vi "VI Icon Browser.vi"() -> ()   [LabVIEW 2011]
panel:
  out "2D VI Icon":picture[][](array[picture])=[[bytes[1002], bytes[798], bytes[222], bytes[318], bytes[558]], [bytes[1512], bytes[537], bytes[1170], bytes[651], bytes[1170]], [bytes[798], bytes[948], bytes[273], bytes[1101], bytes[420]], [bytes[1065], bytes[462], bytes[705], bytes[1380], bytes[798]], [bytes[756], bytes[534], bytes[2118], bytes[714], bytes[798]], [bytes[810], bytes[1230], bytes[798], bytes[1230], bytes[1218]], [bytes[2118], bytes[525], bytes[3102], bytes[1458], bytes[516]], [bytes[1512], bytes[1161], bytes[300], bytes[537], bytes[1662]], [bytes[654], bytes[2298], bytes[798], bytes[798], bytes[1626]], [bytes[732], bytes[1110], bytes[393], bytes[2130], bytes[798]], [bytes[537], bytes[744], bytes[1353], bytes[1488], bytes[345]], [bytes[798], bytes[2379], bytes[222], bytes[273], bytes[798]], [bytes[798], bytes[705], bytes[2382], bytes[525], bytes[1590]], [bytes[390], bytes[0], bytes[0], bytes[0], bytes[0]]]
  out "1D VI Icon":picture[](array[picture])=[bytes[1002], bytes[798], bytes[222], bytes[318], bytes[558], bytes[1512], bytes[537], bytes[1170], bytes[651], bytes[1170], bytes[798], bytes[948], bytes[273], bytes[1101], bytes[420], bytes[1065], bytes[462], bytes[705], bytes[1380], bytes[798], bytes[756], bytes[534], bytes[2118], bytes[714], bytes[798], bytes[810], bytes[1230], bytes[798], bytes[1230], bytes[1218], bytes[2118], bytes[525], bytes[3102], bytes[1458], bytes[516], bytes[1512], bytes[1161], bytes[300], bytes[537], bytes[1662], bytes[654], bytes[2298], bytes[798], bytes[798], bytes[1626], bytes[732], bytes[1110], bytes[393], bytes[2130], bytes[798], bytes[537], bytes[744], bytes[1353], bytes[1488], bytes[345], bytes[798], bytes[2379], bytes[222], bytes[273], bytes[798], bytes[798], bytes[705], bytes[2382], bytes[525], bytes[1590], bytes[390]]
  in  "停止按钮":bool
  in  "VI Icon":string(combo)="操作"
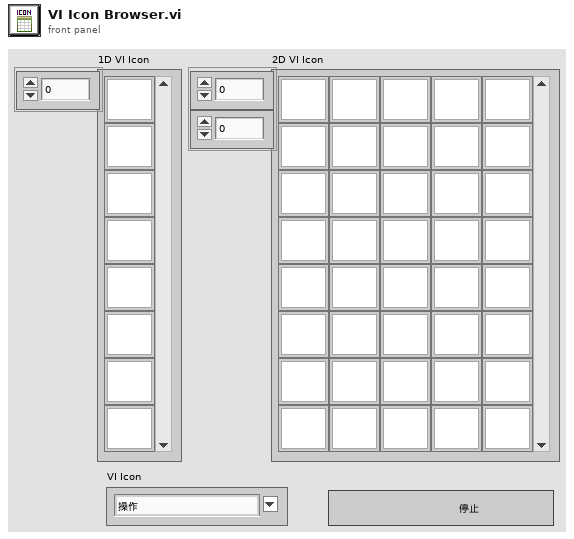
[diagram p1: front panel]
types:
  T1 = typedef "LVBoundsTypeDef.ctl" = cluster{"Width":u32, "Height":u32}
  T2 = typedef "imagedata.ctl" = cluster{"image type":i32, "image depth":i32, "image":u8[], "mask":u8[], "colors":u32[], "Rectangle":cluster{"left":i16, "top":i16, "right":i16, "bottom":i16}}
  T3 = cluster{"left":i16, "top":i16, "right":i16, "bottom":i16}
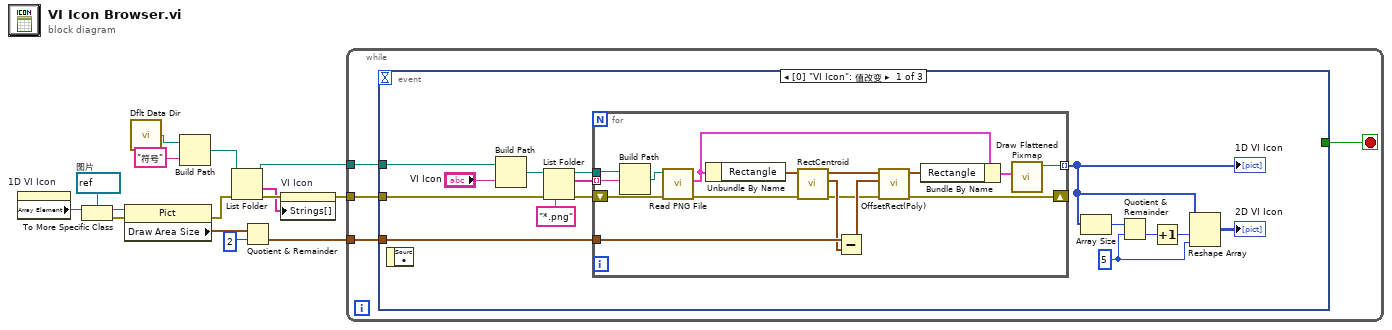
[diagram p0: block diagram]
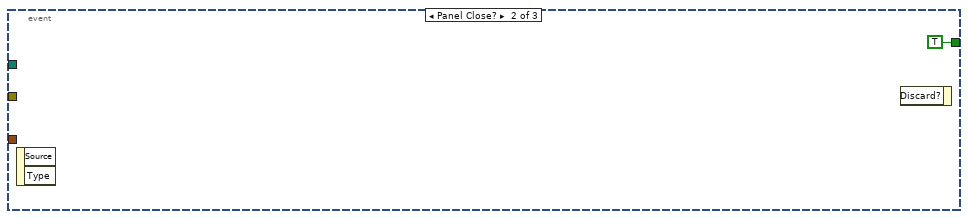
[diagram p2: hidden frame]
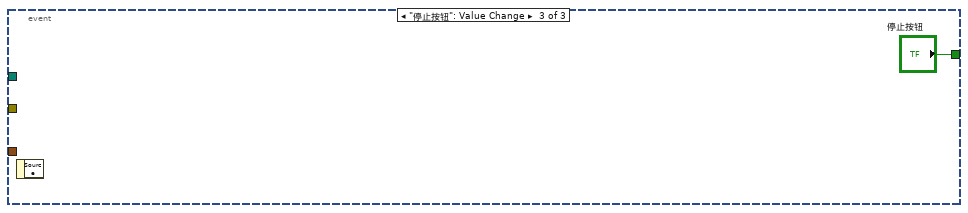
[diagram p3: hidden frame]
diagram:
  w5 = refnum<vi> refnum  # 图片
  n1 = property on="1D VI Icon" class="Arr (严格)"() -> ("Array Element"=w4:refnum<vi>)  [unwired: 2 in, 2 out]
  n2 = To More Specific Class(target class=w5, reference=w4) -> (specific class reference=w6:refnum<vi>, error out=w7:errorcluster)  [unwired: 1 in]
  n3 = property class="Pict"(reference=w6, error in=w7) -> (error out=w1:errorcluster, "Draw Area Size"=w8:T1)  [unwired: 1 out]
  n4 = call <vilib>:"Dflt Data Dir.vi"() -> ("App:Default Data Directory"=w14:path)
  n5 = Build Path(base path=w14, name or relative path="符号" ("名称或相对路径")) -> (appended path=w10:path)
  n6 = List Folder(path=w10, error in=w1) -> (path out=w2:path, folder names=w12:string[], error out=w13:errorcluster)  [unwired: 2 in, 1 out]
  n7 = Quotient & Remainder(x=w8, y=2) -> (floor(x/y)=w3:T1)  [unwired: 1 out]
  n8 = property on="VI Icon" class="CmbBox"(error in=w13, "Strings[]"=w12) -> (error out=w11:errorcluster)  [unwired: 1 in, 1 out]
  n9 = while {
    tunnel: w11 -> [w16]
    tunnel: w2 -> [w18]
    tunnel: w3 -> [w17]
    stop <- w19 stop-if-true
    n10 = event shown="[0] \"VI Icon\": 值改变" {
      selector: _ -> [_ _ _]
      dyn-events: _ -> [_ _ _]
      timeout: _ -> [_ _ _]
      tunnel: [_ TRUE ("停止按钮") "停止按钮"] -> w19
      tunnel: w18 -> [w33 _ _]
      tunnel: w17 -> [w28 _ _]
      tunnel: w16 -> [w21 _ _]
      event "VI Icon": Value Change {
        w22 = 5 ("y")
        n11 = event-data() -> ()  [unwired: 1 in, 1 out]
        n12 = Build Path(base path=w33, name or relative path="VI Icon") -> (appended path=w31:path)
        n13 = List Folder(path=w31, pattern="*.png" ("模式"), error in=w21) -> (path out=w29:path, filenames=w30:string[], error out=w20:errorcluster)  [unwired: 1 in, 1 out]
        n14 = for {
          tunnel: w29 -> [w50]
          tunnel: w30 -> [w49] mode=indexing
          tunnel: [w47] -> w26 mode=indexing
          tunnel: w28 -> [w46]
          shift-right: [w36] -> _
          shift-left: w20 -> [w39]
          n15 = Build Path(base path=w50, name or relative path=w49) -> (appended path=w48:path)
          n16 = call <vilib>:"Read PNG File.vi"("error in (no error)"=w39, "path to PNG file"=w48) -> ("error out"=w38:errorcluster, "image data"=w42:T2)  [unwired: 7 in, 1 out]
          n17 = Unbundle By Name(w42) -> ("Rectangle"=w43:T3)
          n18 = call "RectCentroid.vi"("错误输入"=w38, "Rect In"=w43) -> ("错误输出"=w37:errorcluster, "point"=w45:cluster{"x":i16, "y":i16}, "Rect Out"=w35:T3)  [unwired: 7 in]
          n19 = Subtract(x=w46, y=w45) -> (x-y=w44:T1)
          n20 = call-poly "OffsetRect(Poly).vi"("错误输入"=w37, "point"=w44, "rect"=w35) -> ("错误输出"=w36:errorcluster, "offset rect"=w41:T3)  [unwired: 7 in]
          n21 = Bundle By Name(cluster=w42, "Rectangle"=w41) -> (w40:T2)
          n22 = call <vilib>:"Draw Flattened Pixmap.vi"("image data"=w40) -> ("new picture"=w47:picture)  [unwired: 8 in]
        }
        "1D VI Icon" <- w26
        n23 = Array Size(array=w26) -> (size(s)=w25:i32)
        n24 = Quotient & Remainder(x=w25, y=w22) -> (floor(x/y)=w24:i32)  [unwired: 1 out]
        n25 = Increment(x=w24) -> (x+1=w23:i32)
        n26 = Reshape Array(w26, w23, w22) -> (→"2D VI Icon":picture[][])
      }
      event Panel Close? {
        n27 = event-data() -> ()  [unwired: 1 in, 2 out]
        n28 = event-data() -> ()  [unwired: 2 in, 1 out]
      }
      event "停止按钮": Value Change {
        n29 = event-data() -> ()  [unwired: 1 in, 1 out]
      }
    }
  }
